vi "Neutral_Agilent_E3631A_20151027.vi"(8 "error in (no error)":errorcluster, 10 "Agilent E3631A RefNum":refnum<vi>, 11 "Agilent E3631A Settings":T1={"VISA resource name"="GPIB0::5::INSTR", "Voltage Set (6V max)"=6.0, "Current Set (5A max)"=0.007, "Voltage Set (25V max)"=25.0, "Current Set (1A max)"=0.275, "Voltage Set (-25V max)"=-25.0, "Current Set (1A max)"=0.59, "6V Switch"=FALSE, "+25V Switch"=FALSE, "-25V Switch"=FALSE, "Agilent E3631A Measurements"={"6V Actual Voltage Level (V)"=0.03231557, "6V Actual Current Level (A)"=0.01701259, "25V Actual Voltage Level (V)"=0.4256878, "25V Actual Current Level (A)"=0.2772881, "-25V Actual Current Level (A)"=0.0, "-25V Actual Voltage Level (V)"=0.0}, "Triggered Agilent Settings"={"Trigger \nDelay (s)"=3.0, "Enable +6V Channel"=TRUE, "+6V Current"=0.02, "Enable -25V Channel"=FALSE, "-25V Current"=0.0, "Enable +25V Channel"=TRUE, "+25V Current"=0.275}, "Auto Program Agilent"=FALSE, "Agilent Software Trigger"=FALSE} {"Triggered Agilent Settings"."Trigger \nDelay (s)" min=0.0 max=3600.0 step=1.0 format="%.2f"; "Agilent E3631A Measurements"."-25V Actual Current Level (A)" format="%.3g"; "Agilent E3631A Measurements"."-25V Actual Voltage Level (V)" format="%.3g"; "Agilent E3631A Measurements"."25V Actual Current Level (A)" format="%.3g"; "Agilent E3631A Measurements"."25V Actual Voltage Level (V)" format="%.3g"; "Agilent E3631A Measurements"."6V Actual Current Level (A)" format="%.3g"; "Agilent E3631A Measurements"."6V Actual Voltage Level (V)" format="%.3g"; "Current Set (1A max)" format="%.3g"; "Voltage Set (-25V max)" format="%.3g"; "Current Set (1A max)" format="%.3g"; "Voltage Set (25V max)" format="%.3g"; "Current Set (5A max)" format="%.3g"; "Voltage Set (6V max)" format="%.3g"}) -> (0 "error out":errorcluster={"status"=TRUE, "code"=-1074000000, "source"="Agilent E363X Series.lvlib:Error Query.vi<ERR>\nInstrument reports:\n-222,\"Data out of range\"\r\n+0,\"No error\"\r\n\n\n\n<b>Complete call chain:</b>\r\n     Agilent E363X Series.lvlib:Error Query.vi\r\n     Agilent E363X Series.lvlib:Configure Output.vi\r\n     Neutral_Agilent_E3631A_20151027.vi\r\n     neuKLEIN.vi"})   [LabVIEW 2016]
uses:
  Controls/Agilent E3631A/Settings_Control.ctl
  Controls/Agilent E3631A/Measurement_Indicator.ctl
  Controls/Agilent E3631A/Trigger_Settings.ctl
  Agilent Driver/Agilent E363X Series.lvlib
panel:
  in  "-25V Channel":i32(ring)=3 items=["Channel 1"=1, "Channel 2"=2, "Channel 3"=3]
  in  "+25V Channel":i32(ring)=2 items=["Channel 1"=1, "Channel 2"=2, "Channel 3"=3]
  in  "6V Channel":i32(ring)=1 items=["Channel 1"=1, "Channel 2"=2, "Channel 3"=3]
  # "Since the Agilent is slow to communicate the program will skip programming if the \"Auto Program Agilent\" switch is disabled.  If \"Auto Program\" is enabled the settings to the far left are used to program the Agilent.\n\nAdditionally, the Agilent has an internal software trigger that can a single channel between two current setpoints. The clock is not referenced to the Pulseblaster so be careful with timing when using the Triggered Agilent Settings. To enabled this mode use the \"Agilent Software Trigger\" swithc.\n\nUse the \"Program Agilent\" button to perform a one-time write (with settings on the far left) to avoid having the slow response of the supply during data scans.\n\nNOTE: When setting only current values the program will default to setting the maximum allowed voltage for a given channel."
  # "6V (2017.06.15)\n\nReported Current = \nSet Cur - 0.003A\n\nActual Current = \nSet Cur - 0.0015A"
  # "+25V (2017.06.15)\n\nReported Current = \nSet Cur + 0.002A\n\nActual Current = \nSet Cur + 0.002A"
  # "-25V (2017.06.15)\n\nReported Current = \nSet Cur\n\nActual Current = \nSet Cur"
  # "Beware of the offset in set, reported and actual current from Agilent channels. Below are corrections measured for each channel"
  # "--25V  Measurements"
  # "+25V  Measurements"
  # "6V  Measurements"
  # "-25V Output Settings"
  # "+25V Output Settings"
  # "6V Output Settings"
  # "Since the Agilent is slow to communicate the program will skip programming if the \"Auto Program Agilent\" switch is disabled.  If \"Auto Program\" is enabled the settings to the far left are used to program the Agilent.\n\nAdditionally, the Agilent has an internal software trigger that can a single channel between two current setpoints. The clock is not referenced to the Pulseblaster so be careful with timing when using the Triggered Agilent Settings. To enabled this mode use the \"Agilent Software Trigger\" swithc.\n\nUse the \"Program Agilent\" button to perform a one-time write (with settings on the far left) to avoid having the slow response of the supply during data scans.\n\nNOTE: When setting only current values the program will default to setting the maximum allowed voltage for a given channel."
  # "6V (2017.06.15)\n\nReported Current = \nSet Cur - 0.003A\n\nActual Current = \nSet Cur - 0.0015A"
  # "+25V (2017.06.15)\n\nReported Current = \nSet Cur + 0.002A\n\nActual Current = \nSet Cur + 0.002A"
  # "-25V (2017.06.15)\n\nReported Current = \nSet Cur\n\nActual Current = \nSet Cur"
  # "Beware of the offset in set, reported and actual current from Agilent channels. Below are corrections measured for each channel"
  # "--25V  Measurements"
  # "+25V  Measurements"
  # "6V  Measurements"
  # "-25V Output Settings"
  # "+25V Output Settings"
  # "6V Output Settings"
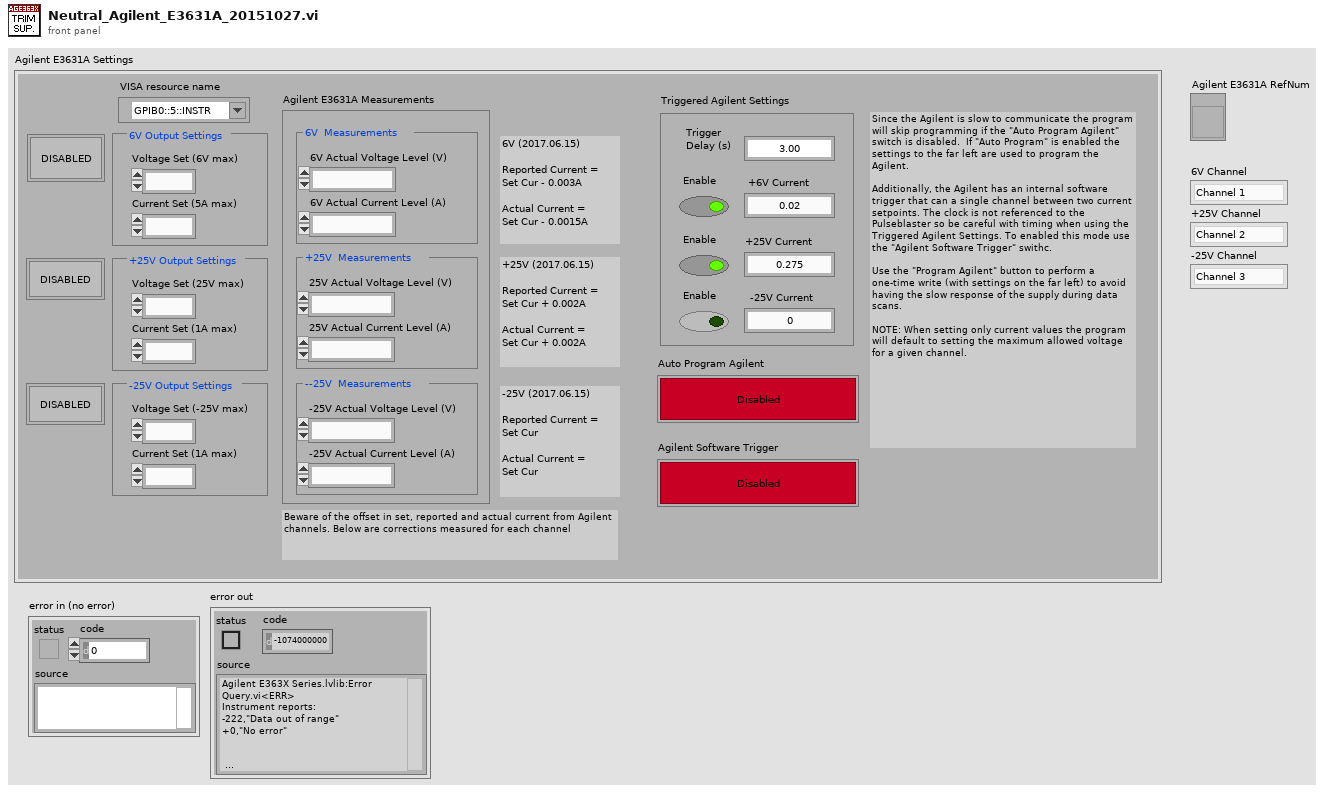
[diagram p1: front panel]
types:
  T1 = typedef "Settings_Control.ctl" = cluster{"VISA resource name":refnum<visa-resource-name>, "Voltage Set (6V max)":dbl, "Current Set (5A max)":dbl, "Voltage Set (25V max)":dbl, "Current Set (1A max)":dbl, "Voltage Set (-25V max)":dbl, "Current Set (1A max)":dbl, "6V Switch":bool, "+25V Switch":bool, "-25V Switch":bool, "Agilent E3631A Measurements":T2, "Triggered Agilent Settings":T3, "Auto Program Agilent":bool, "Agilent Software Trigger":bool}
  T2 = typedef "Measurement_Indicator.ctl" = cluster{"6V Actual Voltage Level (V)":dbl, "6V Actual Current Level (A)":dbl, "25V Actual Voltage Level (V)":dbl, "25V Actual Current Level (A)":dbl, "-25V Actual Current Level (A)":dbl, "-25V Actual Voltage Level (V)":dbl}
  T3 = typedef "Trigger_Settings.ctl" = cluster{"Trigger \nDelay (s)":dbl, "Enable +6V Channel":bool, "+6V Current":dbl, "Enable -25V Channel":bool, "-25V Current":dbl, "Enable +25V Channel":bool, "+25V Current":dbl}
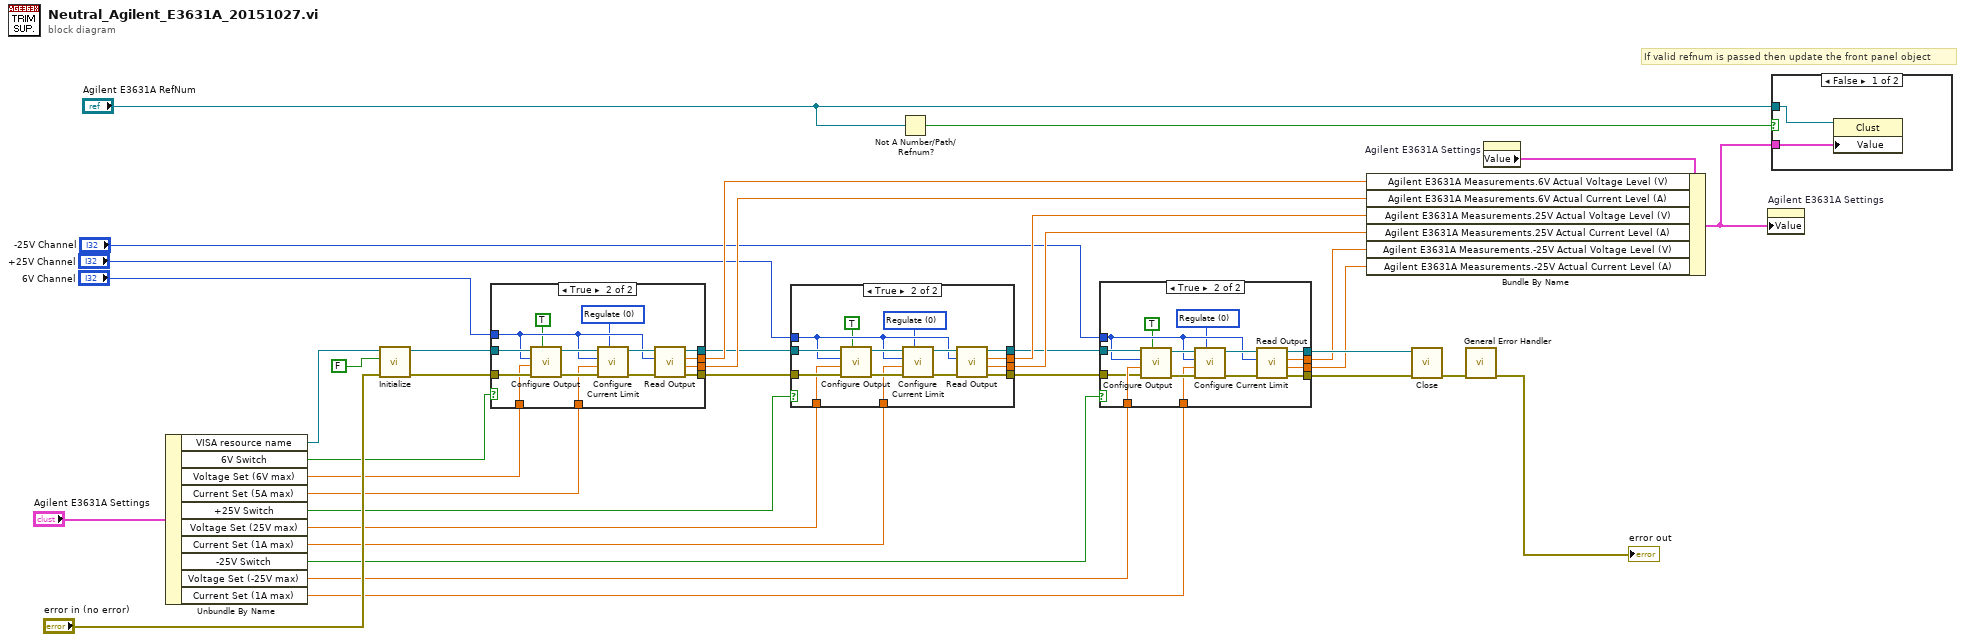
[diagram p0: block diagram]
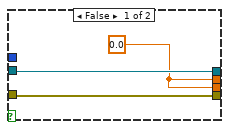
[diagram p2: hidden frame]
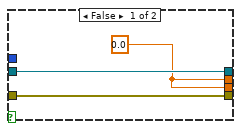
[diagram p3: hidden frame]
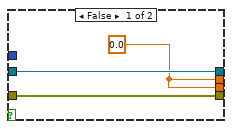
[diagram p4: hidden frame]
diagram:
  # "If valid refnum is passed then update the front panel object"
  n1 = Unbundle By Name("Agilent E3631A Settings") -> ("VISA resource name"=w7:refnum<visa-resource-name>, "6V Switch"=w6:bool, "Voltage Set (6V max)"=w28:dbl, "Current Set (5A max)"=w27:dbl, "+25V Switch"=w4:bool, "Voltage Set (25V max)"=w5:dbl, "Current Set (1A max)"=w21:dbl, "-25V Switch"=w3:bool, "Voltage Set (-25V max)"=w17:dbl, "Current Set (1A max)"=w16:dbl)
  n2 = call "Initialize.vi"("error in (no error)"="error in (no error)", "ID Query? (T: Yes)"=FALSE ("Reset? (T: Yes)"), "VISA resource name"=w7) -> ("error out"=w32:errorcluster, "VISA resource name out"=w34:refnum<visa-resource-name>)  [unwired: 7 in]
  n3 = case shown="True" w6 {
    tunnel: w34 -> [w39 w54]
    tunnel: w32 -> [w38 w53]
    tunnel: "6V Channel" -> [_ w48]
    tunnel: w28 -> [_ w47]
    tunnel: w27 -> [_ w46]
    tunnel: [w37 w45] -> w26
    tunnel: [w37 w44] -> w25
    tunnel: [w38 w43] -> w24
    tunnel: [w39 w42] -> w23
    frame False {
      w37 = 0.0 ("Actual Voltage Level (V)")
    }
    frame True {
      w40 = u16 0 items=["Regulate", "Trip"] ("Behavior (0: Regulate)")
      n4 = call "Configure Output.vi"("Enable Output (T: Enable)"=TRUE, "error in (no error)"=w53, "Voltage Level (0.0 V)"=w47, "Channel (1: Channel 1)"=w48, "VISA resource name"=w54) -> ("error out"=w51:errorcluster, "VISA resource name out"=w52:refnum<visa-resource-name>)  [unwired: 5 in]
      n5 = call "Configure Current Limit.vi"("Behavior (0: Regulate)"=w40, "error in (no error)"=w51, "Current Limit (0.0 A)"=w46, "Channel (1: Channel 1)"=w48, "VISA resource name"=w52) -> ("error out"=w50:errorcluster, "VISA resource name out"=w49:refnum<visa-resource-name>)  [unwired: 5 in]
      n6 = call "Read Output.vi"("error in (no error)"=w50, "Channel (1: Channel 1)"=w48, "VISA resource name"=w49) -> ("error out"=w43:errorcluster, "Actual Current Level (A)"=w44:dbl, "Actual Voltage Level (V)"=w45:dbl, "VISA resource name out"=w42:refnum<visa-resource-name>)  [unwired: 5 in]
    }
  }
  n7 = case shown="True" w4 {
    tunnel: w24 -> [w56 w72]
    tunnel: w23 -> [w57 w69]
    tunnel: "+25V Channel" -> [_ w66]
    tunnel: w21 -> [_ w65]
    tunnel: [w55 w64] -> w20
    tunnel: [w55 w63] -> w19
    tunnel: [w57 w62] -> w15
    tunnel: [w56 w61] -> w14
    tunnel: w5 -> [_ w60]
    frame False {
      w55 = 0.0 ("Actual Voltage Level (V)")
    }
    frame True {
      w58 = u16 0 items=["Regulate", "Trip"] ("Behavior (0: Regulate)")
      n8 = call "Configure Output.vi"("Enable Output (T: Enable)"=TRUE, "error in (no error)"=w72, "Voltage Level (0.0 V)"=w60, "Channel (1: Channel 1)"=w66, "VISA resource name"=w69) -> ("error out"=w71:errorcluster, "VISA resource name out"=w68:refnum<visa-resource-name>)  [unwired: 5 in]
      n9 = call "Configure Current Limit.vi"("Behavior (0: Regulate)"=w58, "error in (no error)"=w71, "Current Limit (0.0 A)"=w65, "Channel (1: Channel 1)"=w66, "VISA resource name"=w68) -> ("error out"=w70:errorcluster, "VISA resource name out"=w67:refnum<visa-resource-name>)  [unwired: 5 in]
      n10 = call "Read Output.vi"("error in (no error)"=w70, "Channel (1: Channel 1)"=w66, "VISA resource name"=w67) -> ("error out"=w61:errorcluster, "Actual Current Level (A)"=w63:dbl, "Actual Voltage Level (V)"=w64:dbl, "VISA resource name out"=w62:refnum<visa-resource-name>)  [unwired: 5 in]
    }
  }
  n11 = Not A Number/Path/Refnum?(number/path/refnum="Agilent E3631A RefNum") -> (NaN/Path/Refnum?=w18:bool)
  n12 = case shown="True" w3 {
    tunnel: w17 -> [_ w86]
    tunnel: w16 -> [_ w85]
    tunnel: w15 -> [w74 w84]
    tunnel: w14 -> [w75 w83]
    tunnel: [w74 w82] -> w13
    tunnel: [w75 w81] -> w12
    tunnel: [w73 w80] -> w11
    tunnel: [w73 w79] -> w10
    tunnel: "-25V Channel" -> [_ w78]
    frame False {
      w73 = 0.0 ("Actual Voltage Level (V)")
    }
    frame True {
      w76 = u16 0 items=["Regulate", "Trip"] ("Behavior (0: Regulate)")
      n13 = call "Configure Output.vi"("Enable Output (T: Enable)"=TRUE, "error in (no error)"=w83, "Voltage Level (0.0 V)"=w86, "Channel (1: Channel 1)"=w78, "VISA resource name"=w84) -> ("error out"=w90:errorcluster, "VISA resource name out"=w88:refnum<visa-resource-name>)  [unwired: 5 in]
      n14 = call "Configure Current Limit.vi"("Behavior (0: Regulate)"=w76, "error in (no error)"=w90, "Current Limit (0.0 A)"=w85, "Channel (1: Channel 1)"=w78, "VISA resource name"=w88) -> ("error out"=w89:errorcluster, "VISA resource name out"=w87:refnum<visa-resource-name>)  [unwired: 5 in]
      n15 = call "Read Output.vi"("error in (no error)"=w89, "Channel (1: Channel 1)"=w78, "VISA resource name"=w87) -> ("error out"=w81:errorcluster, "Actual Current Level (A)"=w79:dbl, "Actual Voltage Level (V)"=w80:dbl, "VISA resource name out"=w82:refnum<visa-resource-name>)  [unwired: 5 in]
    }
  }
  n16 = call "Close.vi"("error in (no error)"=w12, "VISA resource name"=w13) -> ("error out"=w33:errorcluster)  [unwired: 9 in]
  n17 = call <vilib>:"General Error Handler.vi"("error in (no error)"=w33) -> ("error out"=→"error out":errorcluster)  [unwired: 10 in, 4 out]
  n18 = property on="Agilent E3631A Settings" class="Clust (strict)"() -> ("Value"=w35:T1)  [unwired: 2 in, 2 out]
  n19 = Bundle By Name(cluster=w35, "Agilent E3631A Measurements.6V Actual Voltage Level (V)"=w26, "Agilent E3631A Measurements.6V Actual Current Level (A)"=w25, "Agilent E3631A Measurements.25V Actual Voltage Level (V)"=w20, "Agilent E3631A Measurements.25V Actual Current Level (A)"=w19, "Agilent E3631A Measurements.-25V Actual Voltage Level (V)"=w11, "Agilent E3631A Measurements.-25V Actual Current Level (A)"=w10) -> (w1:T1)
  n20 = property on="Agilent E3631A Settings" class="Clust (strict)"("Value"=w1) -> ()  [unwired: 2 in, 2 out]
  n21 = case shown="False" w18 {
    tunnel: "Agilent E3631A RefNum" -> [w92 _]
    tunnel: w1 -> [w91 _]
    frame False {
      n22 = property on="Property Node" class="Clust"(reference=w92, "Value"=w91) -> ()  [unwired: 1 in, 2 out]
    }
    frame True {
    }
  }
